vi "stringArraryFilter.vi"(0 "inputFeature":string[](array[string]), 5 "stringLength":i32, 7 "stringFilterBegin":string, 9 "stringFilterEnd":string) -> (4 "outputFeature":string[](array[string]))   [LabVIEW 2018]
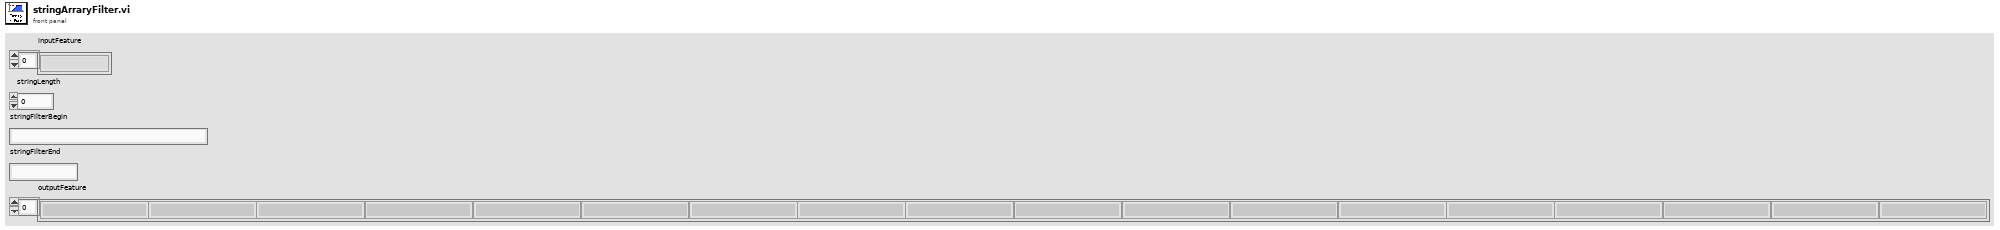
[diagram p1: front panel]
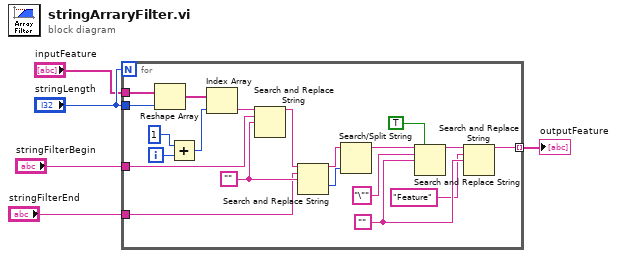
[diagram p0: block diagram]
diagram:
  n1 = for {
    N: "stringLength" -> [_]
    tunnel: "inputFeature" -> [w12]
    tunnel: "stringFilterBegin" -> [w16]
    tunnel: "stringFilterEnd" -> [w15]
    tunnel: "stringLength" -> [w13]
    tunnel: [w7] -> w5 mode=indexing
    i -> [w25]
    w9 = ""
    w17 = ""
    n2 = Reshape Array(w12, w13) -> (w11:string[])
    n3 = Add(x=1, y=w25) -> (x+y=w14:i32)
    n4 = Index Array(array=w11, index=w14) -> (element=w10:string)
    n5 = Search and Replace String(input string=w10, search string=w16, replace string=w17) -> (result string=w18:string)  [unwired: 5 in, 3 out]
    n6 = Search and Replace String(input string=w18, search string=w15, replace string=w17) -> (result string=w20:string, offset past replacement=w19:i32)  [unwired: 5 in, 2 out]
    n7 = Search/Split String(string=w20, offset (0)=w19) -> (substring before match=w21:string)  [unwired: 1 in, 2 out]
    n8 = Search and Replace String(replace all?=TRUE ("replace all? (F)"), input string=w21, search string="\"", replace string=w9) -> (result string=w8:string)  [unwired: 4 in, 3 out]
    n9 = Search and Replace String(input string=w8, search string="Feature" ("replace string (\"\")"), replace string=w9) -> (result string=w7:string)  [unwired: 5 in, 3 out]
  }
  "outputFeature" <- w5
